vi "EOL NVH Inputs Controls Buffer 2.0.vi"(6 "NVH Configuration":T1, 8 "Error in":string[][](array[string]), 9 "NVH Inputs":bool[](array[boolean]), 10 "NVHK Inputs Control":T3[](array[typedef]), 11 "Mode":T2=enum."Read") -> (0 "Error out":string[][](array[string]), 1 "NVH All Inputs":bool[](array[boolean]), 2 "NVH Single Input":bool, 3 "NVH Inputs Out":bool[](array[boolean]), 4 "NVH_PartNumber_Echo":u16)   [LabVIEW 2018]
uses:
  02.Type Def's/NVH Digital Input.ctl
  02.Type Def's/NVH Mode Control 2.0.ctl
  02.Type Def's/station nvh config.ctl
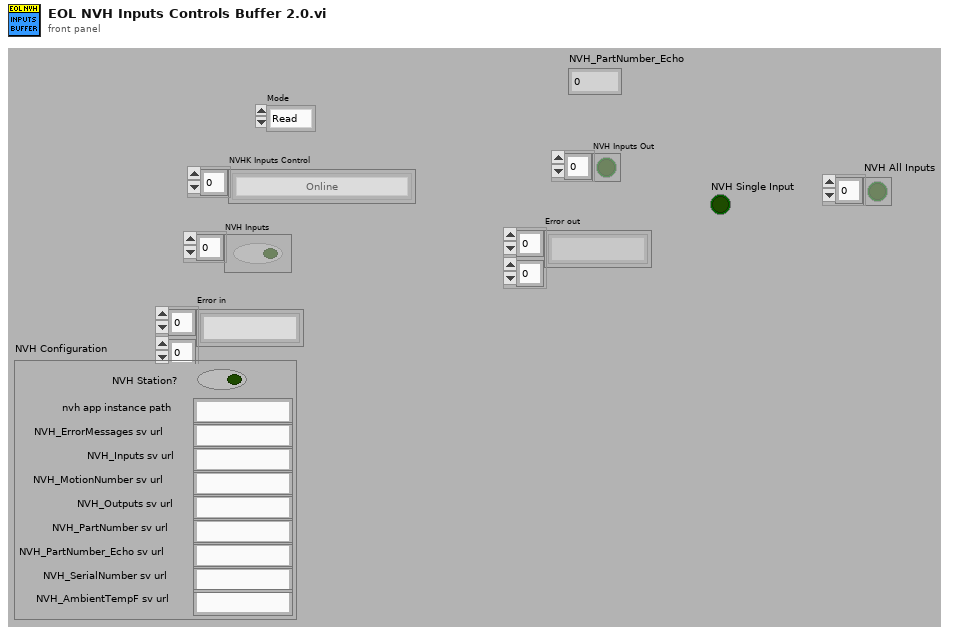
[diagram p1: front panel]
types:
  T1 = typedef "station nvh config.ctl" = cluster{"NVH Station?":bool, "nvh app instance path":string, "NVH_ErrorMessages sv url":string, "NVH_Inputs sv url":string, "NVH_MotionNumber sv url":string, "NVH_Outputs sv url":string, "NVH_PartNumber sv url":string, "NVH_PartNumber_Echo sv url":string, "NVH_SerialNumber sv url":string, "NVH_AmbientTempF sv url":string}
  T2 = typedef "NVH Mode Control 2.0.ctl" = enum16{"Init", "Write", "Write String", "Read", "Write Part Number", "Write Motion Number", "Write Ambient TempF"}
  T3 = typedef "NVH Digital Input.ctl" = enum16{"Online", "Pass", "Fail", "Testing", "Ready for Model", "Error Bit 1", "Error Bit 2", "Error Bit 3", "Failure Bit 1", "Failure Bit 2", "Failure Bit 3", "Failure Bit 4", "Echo Bit 1", "Echo Bit 2", "Echo Bit 3", "Echo Bit 4", "Serial Number Read Ok", "Ready for Serrial Number"}
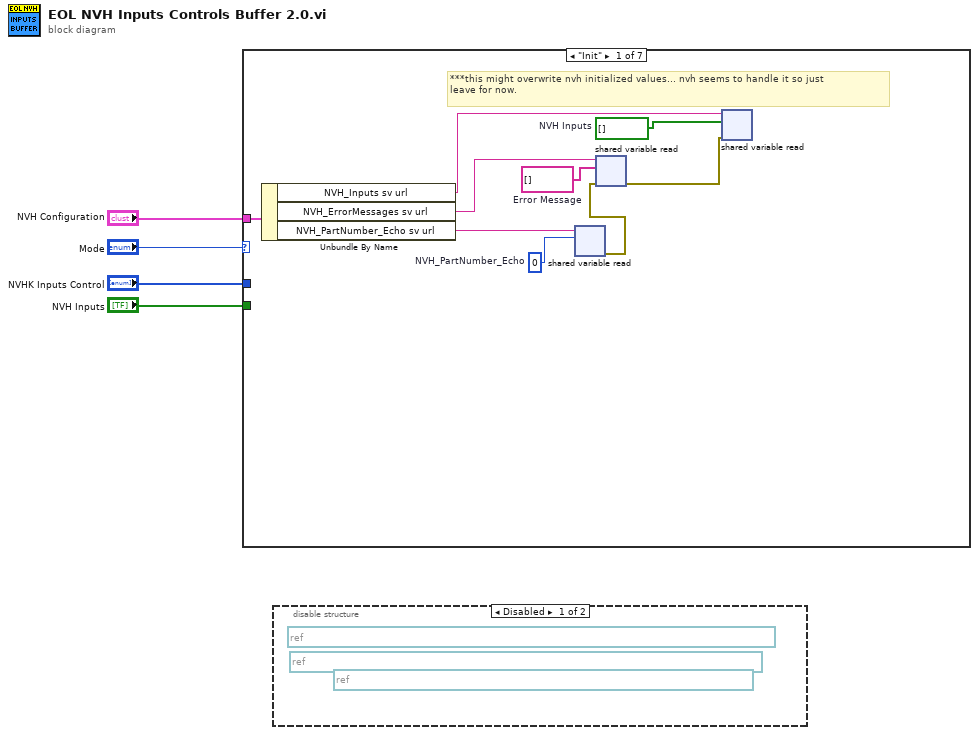
[diagram p0: block diagram]
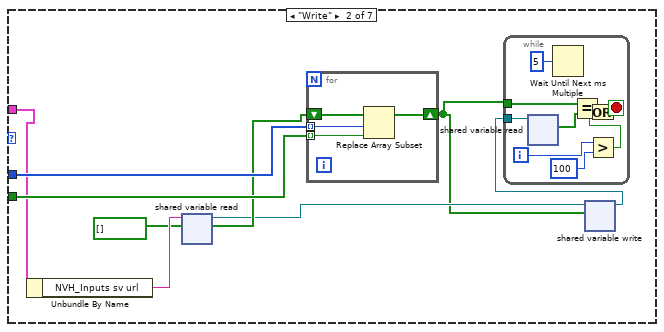
[diagram p2: hidden frame]
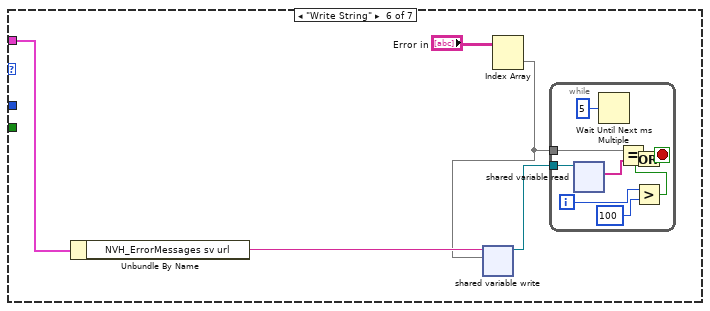
[diagram p6: hidden frame]
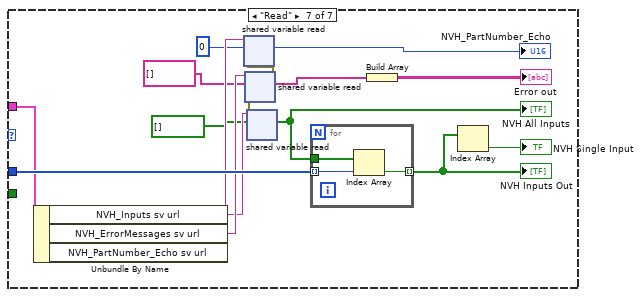
[diagram p7: hidden frame]
diagram:
  n1 = case shown="\"Init\"" "Mode" {
    tunnel: "NVHK Inputs Control" -> [_ w22 _ _ _ _ w64]
    tunnel: "NVH Inputs" -> [_ w21 _ _ _ _ _]
    tunnel: "NVH Configuration" -> [w13 w18 _ _ _ w37 w58]
    frame "Init" {
      w7 = u16 0  # NVH_PartNumber_Echo
      w9 = string[] []  # Error Message
      w11 = bool[] []  # NVH Inputs
      # "***this might overwrite nvh initialized values... nvh seems to handle it so just\nleave for now."
      n2 = Unbundle By Name(w13) -> ("NVH_Inputs sv url"=w12:string, "NVH_ErrorMessages sv url"=w10:string, "NVH_PartNumber_Echo sv url"=w8:string)
      n3 = shared-variable-read(w8, w7) -> (w6:errorcluster)  [unwired: 1 in, 3 out]
      n4 = shared-variable-read(w10, w6, w9) -> (w5:errorcluster)  [unwired: 3 out]
      n5 = shared-variable-read(w12, w5, w11) -> ()  [unwired: 4 out]
    }
    frame "Write" {
      n6 = Unbundle By Name(w18) -> ("NVH_Inputs sv url"=w20:string)
      n7 = shared-variable-read(w20, bool[] [] ("NVH Inputs")) -> (w15:refnum<k21>, w17:bool[])  [unwired: 1 in, 2 out]
      n8 = for {
        shift-right: [w32] -> w14
        shift-left: w17 -> [w35]
        tunnel: w22 -> [w34] mode=indexing
        tunnel: w21 -> [w33] mode=indexing
        n9 = Replace Array Subset(array=w35, new element=w33, index=w34) -> (w32:bool[])
      }
      n10 = shared-variable-write(w15, w14) -> (w16:refnum<k21>)  [unwired: 1 in, 1 out]
      n11 = while {
        tunnel: w16 -> [w31]
        tunnel: w14 -> [w28]
        i -> [w25]
        stop <- w26 stop-if-true
        n12 = shared-variable-read(w31) -> (w29:bool[])  [unwired: 1 in, 3 out]
        n13 = Wait Until Next ms Multiple(millisecond multiple=u32 5) -> ()  [unwired: 1 out]
        n14 = Equal?(x=w28, y=w29) -> (x = y?=w27:bool)
        n15 = Greater?(x=w25, y=100) -> (0:w23:bool)
        n16 = Or(x=w27, y=w23) -> (x .or. y?=w26:bool)
      }
    }
    frame "Write Motion Number" {
    }
    frame "Write Ambient TempF" {
    }
    frame "Write Part Number" {
    }
    frame "Write String" {
      n17 = Unbundle By Name(w37) -> ("NVH_ErrorMessages sv url"=w38:string)
      n18 = Index Array(array="Error in") -> (element=w36:string[])  [unwired: 2 in]
      n19 = shared-variable-write(w38, w36) -> (w39:refnum<k21>)  [unwired: 1 in, 1 out]
      n20 = while {
        tunnel: w39 -> [w49]
        tunnel: w36 -> [w46]
        i -> [w43]
        stop <- w44 stop-if-true
        n21 = shared-variable-read(w49) -> (w47:string[])  [unwired: 1 in, 3 out]
        n22 = Wait Until Next ms Multiple(millisecond multiple=u32 5) -> ()  [unwired: 1 out]
        n23 = Equal?(x=w46, y=w47) -> (x = y?=w45:bool)
        n24 = Greater?(x=w43, y=100) -> (0:w41:bool)
        n25 = Or(x=w45, y=w41) -> (x .or. y?=w44:bool)
      }
    }
    frame "Read" {
      n26 = Unbundle By Name(w58) -> ("NVH_Inputs sv url"=w53:string, "NVH_ErrorMessages sv url"=w55:string, "NVH_PartNumber_Echo sv url"=w57:string)
      n27 = shared-variable-read(w53, bool[] [] ("NVH Inputs")) -> (w51:errorcluster, w62:bool[])  [unwired: 1 in, 2 out]
      "NVH All Inputs" <- w62
      n28 = shared-variable-read(w55, w51, string[] [] ("subarray")) -> (w50:errorcluster, w61:string[])  [unwired: 2 out]
      n29 = shared-variable-read(w57, w50, u16 0 ("data out")) -> (→"NVH_PartNumber_Echo":u16)  [unwired: 3 out]
      n30 = for {
        tunnel: w64 -> [w67] mode=indexing
        tunnel: w62 -> [w68]
        tunnel: [w66] -> w63 mode=indexing
        n31 = Index Array(array=w68, index=w67) -> (element=w66:bool)
      }
      "NVH Inputs Out" <- w63
      n32 = Build Array(w61) -> (→"Error out":string[][])
      n33 = Index Array(array=w63) -> (element=→"NVH Single Input":bool)  [unwired: 1 in]
    }
  }
  n34 = disable-structure shown="Disabled" {
    frame Disabled {
      (unwired) refnum<k21> "ni.var.psp://My Computer/NVH Communication Library/NVH_Inputs" ("shared variable refnum in")
      (unwired) refnum<k21> "ni.var.psp://My Computer/NVH Communication Library/NVH_ErrorMessages" ("shared variable refnum in")
      (unwired) refnum<k21> "ni.var.psp://My Computer/NVH Communication Library/NVH_PartNumber_Echo" ("shared variable refnum in")
    }
    frame Enabled {
    }
  }
